vi "OP600ZP_Param_Conf.vi"(8 "errin":errorcluster, 10 "Chaîne":string, 11 "pathin":path) -> (0 "errout":errorcluster, 3 "VISA OUT":T1)   [LabVIEW 2020]
uses:
  <vilib>/Utility/config.llb/Read Key (String).vi
  <vilib>/Utility/config.llb/NI_LVConfig.lvlib
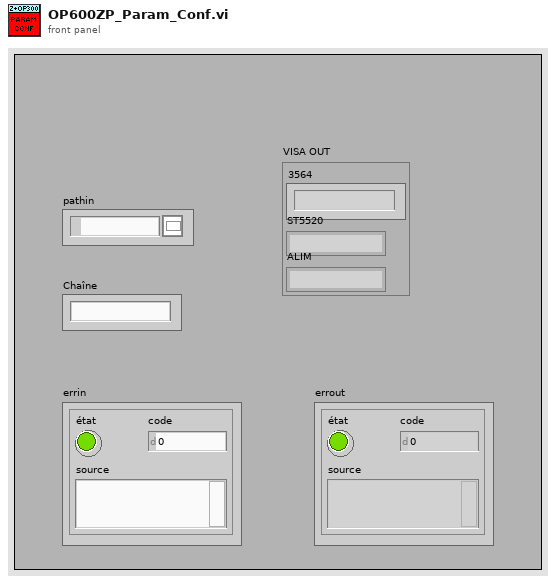
[diagram p1: front panel]
types:
  T1 = cluster{"3564":string, "ST5520":string, "ALIM":string}
  T2 = typedef "NI_LVConfig.lvlib/Config Data RefNum.ctl" = refnum<k1>
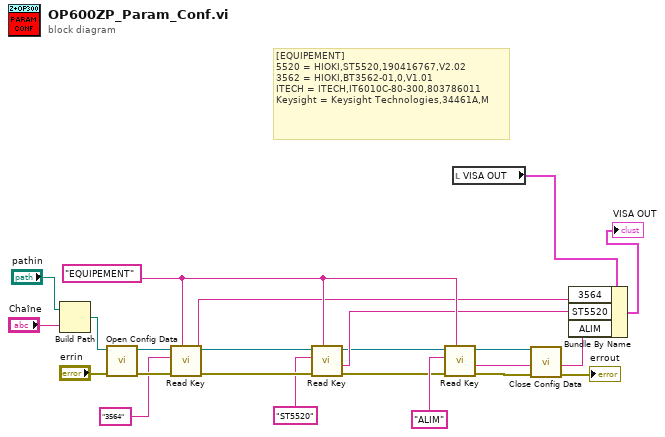
[diagram p0: block diagram]
diagram:
  w7 = "EQUIPEMENT" ("section")
  # "[EQUIPEMENT]\n5520 = HIOKI,ST5520,190416767,V2.02\n3562 = HIOKI,BT3562-01,0,V1.01\nITECH = ITECH,IT6010C-80-300,803786011\nKeysight = Keysight Technologies,34461A,M"
  n1 = Build Path(base path="pathin", name or relative path="Chaîne") -> (appended path=w19:path)
  n2 = call <vilib>:"Open Config Data.vi"("error in (no error)"="errin", "configuration file path"=w19) -> ("error out"=w21:errorcluster, "refnum"=w22:T2)  [unwired: 7 in, 1 out]
  n3 = call-poly <vilib>:"Read Key.vi"("section"=w7, "error in (no error)"=w21, "key"="3564", "refnum"=w22) -> ("error out"=w16:errorcluster, "value"=w5:string, "refnum out"=w18:T2)  [unwired: 4 in, 1 out]
  n4 = call-poly <vilib>:"Read Key.vi"("section"=w7, "error in (no error)"=w16, "key"="ST5520", "refnum"=w18) -> ("error out"=w2:errorcluster, "value"=w4:string, "refnum out"=w3:T2)  [unwired: 4 in, 1 out]
  n5 = call-poly <vilib>:"Read Key.vi"("section"=w7, "error in (no error)"=w2, "key"="ALIM", "refnum"=w3) -> ("error out"=w1:errorcluster, "value"=w6:string, "refnum out"=w9:T2)  [unwired: 4 in, 1 out]
  n6 = local read "VISA OUT"() -> (w12:T1)
  n7 = call <vilib>:"Close Config Data.vi"("error in (no error)"=w1, "refnum"=w9) -> ("error out"=→"errout":errorcluster)  [unwired: 8 in, 1 out]
  n8 = Bundle By Name(cluster=w12, "3564"=w5, "ST5520"=w4, "ALIM"=w6) -> (→"VISA OUT":T1)
